vi "Watlow Global.vi"(7 "Write (F)":bool, 9 "Watlow is F4T?":bool, 10 "3 Pump Tank":bool, 11 "Watlow Present":bool) -> (1 "Watlow is F4T? OUT":bool, 2 "3 Pump Tank OUT":bool, 3 "Watlow Present OUT":bool)   [LabVIEW 2013]
panel:
  out "Watlow Present":bool
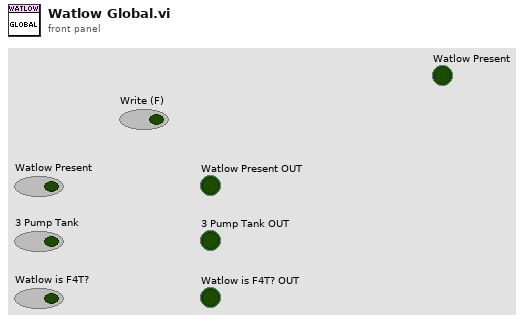
[diagram p1: front panel]
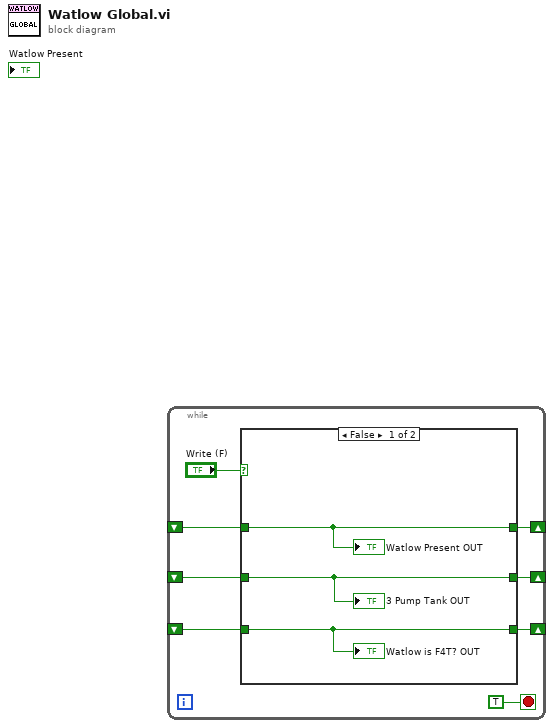
[diagram p0: block diagram]
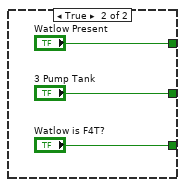
[diagram p2: hidden frame]
diagram:
  n1 = while {
    shift-right: [w6] -> _
    shift-left: _ -> [w5]
    shift-right: [w4] -> _
    shift-left: _ -> [w3]
    shift-right: [w2] -> _
    shift-left: _ -> [w1]
    stop <- TRUE stop-if-true
    n2 = case shown="False" "Write (F)" {
      tunnel: [w11 "Watlow Present"] -> w6
      tunnel: w5 -> [w11 _]
      tunnel: [w10 "Watlow is F4T?"] -> w4
      tunnel: w3 -> [w10 _]
      tunnel: [w9 "3 Pump Tank"] -> w2
      tunnel: w1 -> [w9 _]
      frame False {
        "Watlow Present OUT" <- w11
        "Watlow is F4T? OUT" <- w10
        "3 Pump Tank OUT" <- w9
      }
      frame True {
      }
    }
  }
